vi "motioncontroller.vi"(3 "Error in x":errorcluster, 5 "VISA IN x":refnum<visa-resource-name>) -> (0 "Error out x":errorcluster, 2 "VISA OUT x":refnum<visa-resource-name>)   [LabVIEW 2016]
uses:
  <vilib>/Instr/_visa.llb/VISA Flush IO Buffer Mask.ctl
  <vilib>/Instr/_visa.llb/VISA Configure Serial Port (Instr).vi
panel:
  in  "Dy (mm)":dbl
  in  "Dx (mm)":dbl
  in  "y (mm)":dbl
  in  "x (mm)":dbl
  out "string to y (hex)":string
  in  "command to y":string
  out "VISA OUT y":refnum<visa-resource-name>
  out "Error out y":errorcluster
  out "answer from y (hex)":string
  in  "VISA IN y":refnum<visa-resource-name>
  in  "Error in y":errorcluster
  out "string to x (hex)":string
  in  "command to x":string
  in  "SHIFT":bool
  in  "MOVE":bool
  out "answer from x (hex)":string
  in  "SEND":bool
  in  "EXIT":bool
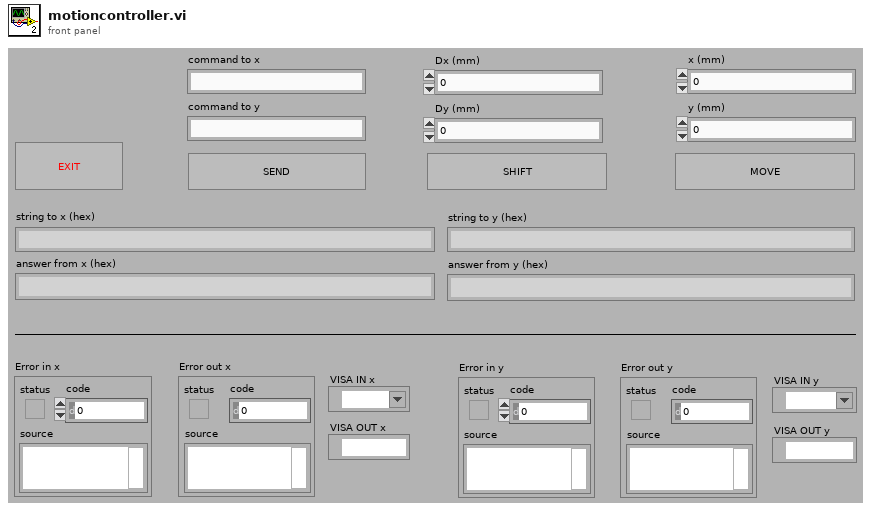
[diagram p1: front panel]
types:
  T1 = typedef "VISA Flush IO Buffer Mask.ctl" = u16
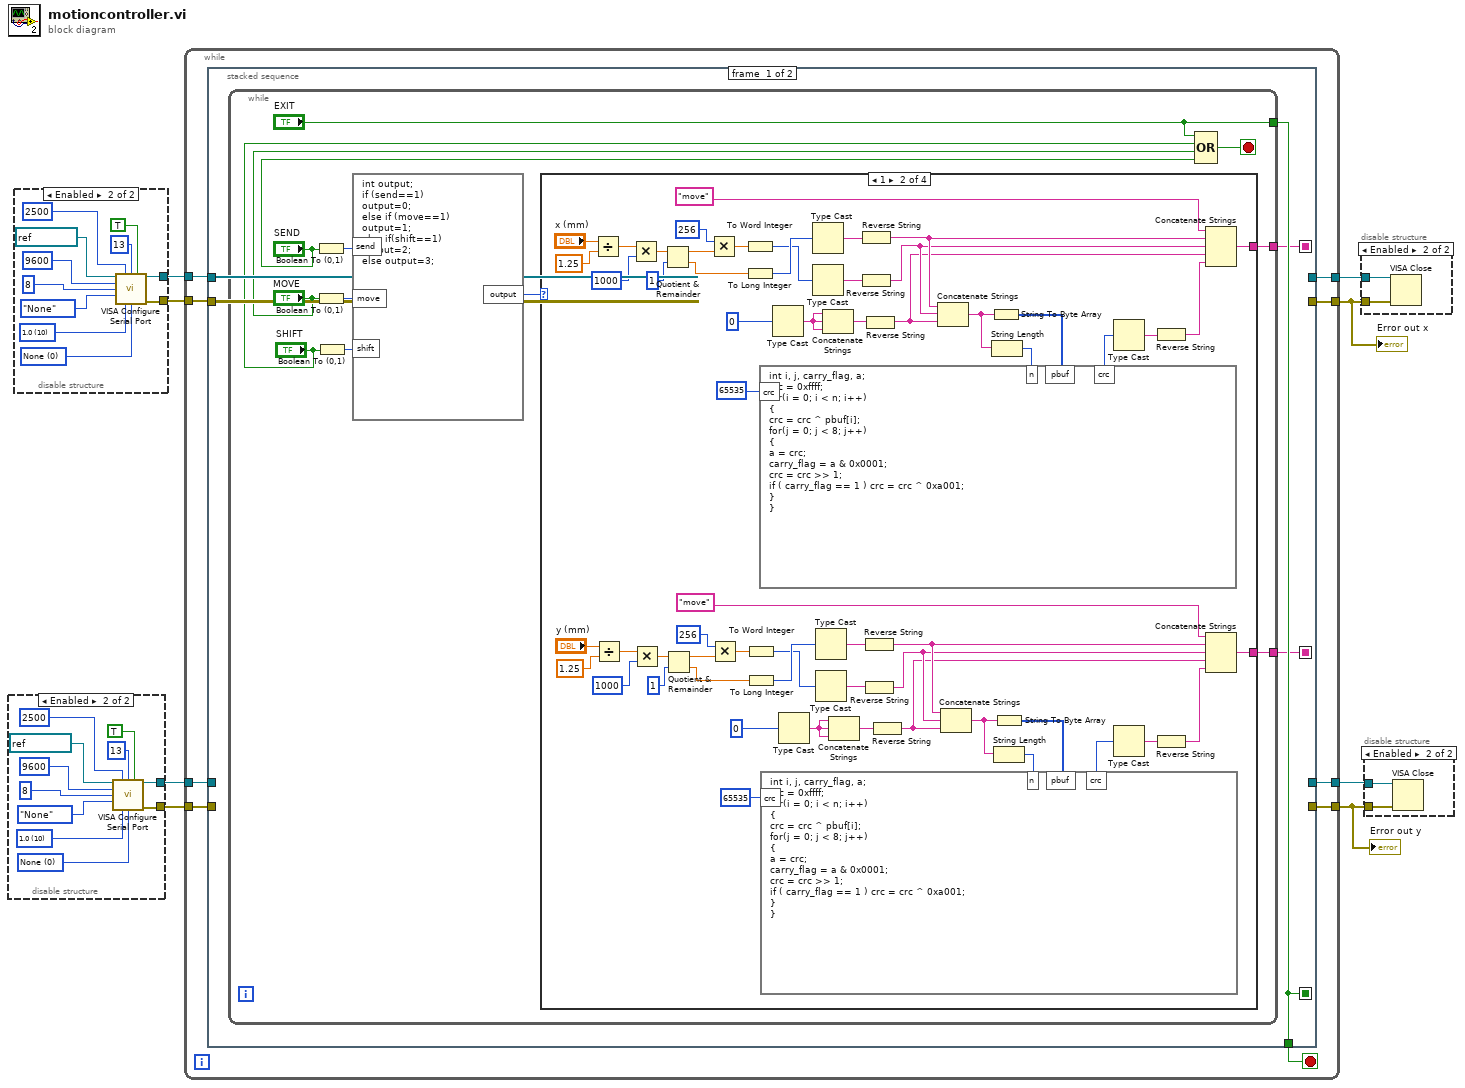
[diagram p0: block diagram]
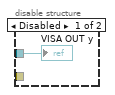
[diagram p2: hidden frame]
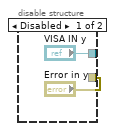
[diagram p3: hidden frame]
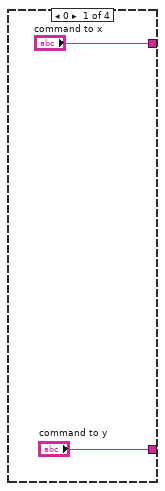
[diagram p4: hidden frame]
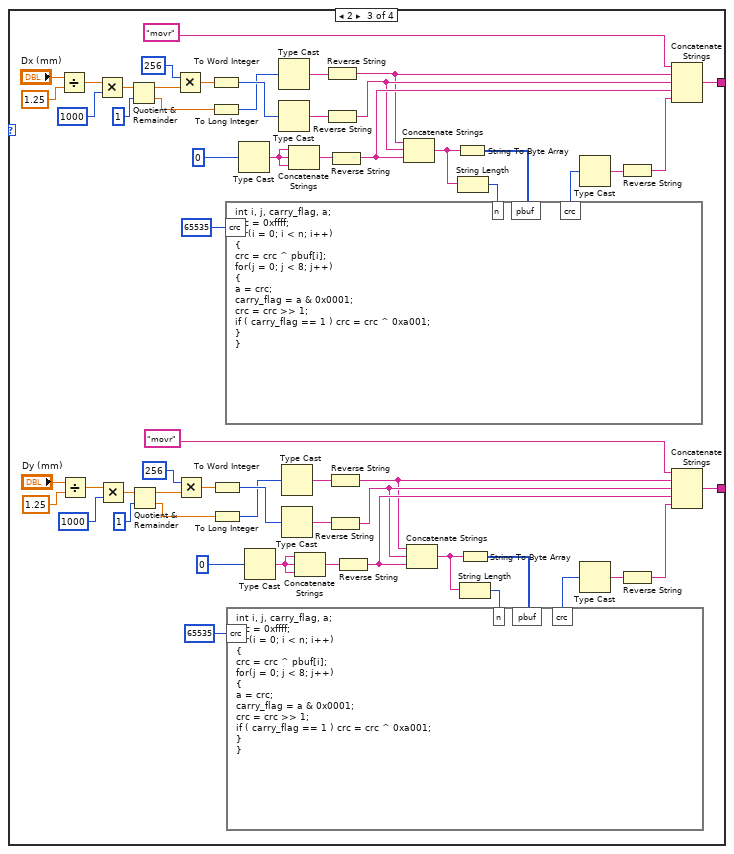
[diagram p5: hidden frame]
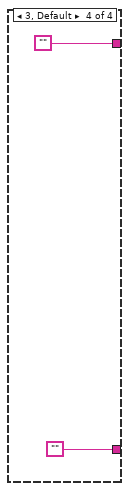
[diagram p6: hidden frame]
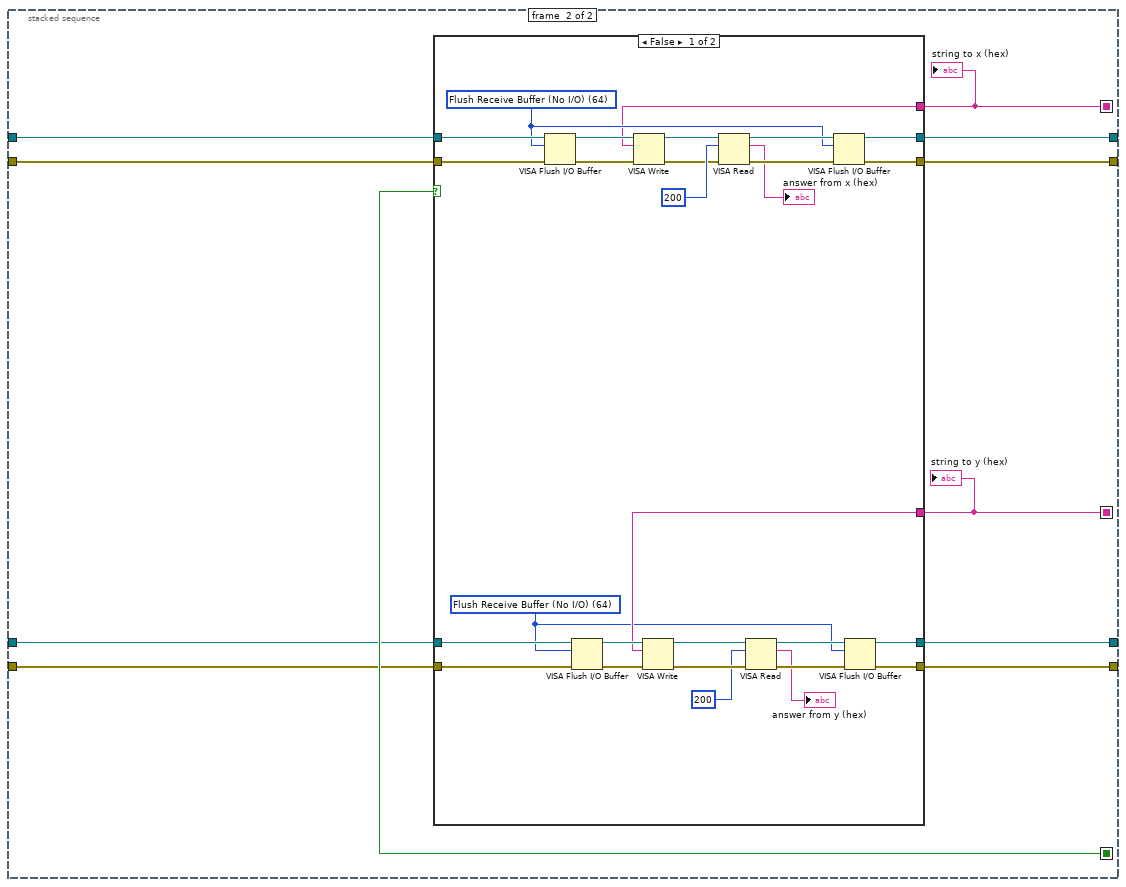
[diagram p7: hidden frame]
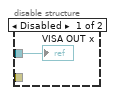
[diagram p9: hidden frame]
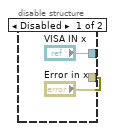
[diagram p10: hidden frame]
diagram:
  n1 = disable-structure shown="Enabled" {
    disable-tunnel: ["VISA IN y" w13] -> w6
    disable-tunnel: ["Error in y" w12] -> w5
    frame Disabled {
    }
    frame Enabled {
      w18 = u16 0 items=["None", "XON/XOFF", "RTS/CTS", "XON/XOFF & RTS/CTS", "DTR/DSR", "XON/XOFF & DTR/DSR"] ("flow control (0:none)")
      w17 = u16 10 items=["1.0"=10, "1.5"=15, "2.0"=20] ("stop bits (10: 1 bit)")
      n2 = call-poly "VISA Configure Serial Port"("VISA resource name"=refnum<visa-resource-name> "COM4" ("VISA resource name y"), "timeout (10sec)"=u32 2500, "termination char\n(0xA = '\\n' = LF)"=u8 13 ("termination char\n(0xA = '\\n' = LF)"), "Enable Termination\nChar (T)"=TRUE ("Enable Termination\nChar (T)"), "baud rate (9600)"=u32 9600, "data bits (8)"=u16 8, "parity (0:none)"=enum16{"None", "Odd", "Even", "Mark", "Space"}."None", "stop bits (10: 1 bit)"=w17, "flow control (0:none)"=w18) -> ("VISA resource name out"=w13:refnum<visa-resource-name>, "error out"=w12:errorcluster)  [unwired: 1 in, 4 out]
    }
  }
  n3 = disable-structure shown="Enabled" {
    disable-tunnel: ["VISA IN x" w26] -> w8
    disable-tunnel: ["Error in x" w25] -> w7
    frame Disabled {
    }
    frame Enabled {
      w31 = u16 0 items=["None", "XON/XOFF", "RTS/CTS", "XON/XOFF & RTS/CTS", "DTR/DSR", "XON/XOFF & DTR/DSR"] ("flow control (0:none)")
      w30 = u16 10 items=["1.0"=10, "1.5"=15, "2.0"=20] ("stop bits (10: 1 bit)")
      n4 = call-poly "VISA Configure Serial Port"("VISA resource name"=refnum<visa-resource-name> "COM3" ("VISA resource name x"), "timeout (10sec)"=u32 2500, "termination char\n(0xA = '\\n' = LF)"=u8 13 ("termination char\n(0xA = '\\n' = LF)"), "Enable Termination\nChar (T)"=TRUE ("Enable Termination\nChar (T)"), "baud rate (9600)"=u32 9600, "data bits (8)"=u16 8, "parity (0:none)"=enum16{"None", "Odd", "Even", "Mark", "Space"}."None", "stop bits (10: 1 bit)"=w30, "flow control (0:none)"=w31) -> ("VISA resource name out"=w26:refnum<visa-resource-name>, "error out"=w25:errorcluster)  [unwired: 1 in, 4 out]
    }
  }
  n5 = while {
    tunnel: w8 -> [w43]
    tunnel: w7 -> [w42]
    tunnel: w6 -> [w40]
    tunnel: w5 -> [w39]
    tunnel: [w38] -> w4
    tunnel: [w37] -> w3
    tunnel: [w36] -> w1
    tunnel: [w35] -> w2
    stop <- w41 stop-if-true
    n6 = stacked-sequence {
      seq-local: [w46 _] -> [_ w184]
      seq-local: [w44 _] -> [_ w178]
      seq-local: [w45 _] -> [_ w179]
      tunnel: [_ w188] -> w36
      tunnel: w43 -> [_ w187]
      tunnel: w42 -> [_ w186]
      tunnel: [_ w185] -> w35
      tunnel: [w46 _] -> w41
      tunnel: w40 -> [_ w183]
      tunnel: w39 -> [_ w182]
      tunnel: [_ w181] -> w38
      tunnel: [_ w180] -> w37
      frame #0 {
        n7 = while {
          tunnel: ["EXIT"] -> w46
          tunnel: [w48] -> w44
          tunnel: [w47] -> w45
          stop <- w53 stop-if-true
          n8 = Boolean To (0,1)(Boolean="SEND") -> (0, 1=w56:i16)
          n9 = Boolean To (0,1)(Boolean="MOVE") -> (0, 1=w55:i16)
          n10 = Boolean To (0,1)(Boolean="SHIFT") -> (0, 1=w54:i16)
          n11 = formula code="int output;\nif (send==1)\noutput=0;\nelse if (move==1)\noutput=1;\nelse if(shift==1)\noutput=2;\nelse output=3;"("send"=w56, "move"=w55, "shift"=w54) -> ("output"=w57:i32)
          n12 = case shown="1" w57 {
            tunnel: ["command to x" w60 w119 ""] -> w48
            tunnel: ["command to y" w61 w118 ""] -> w47
            frame 0 {
            }
            frame 1 {
              n13 = Divide(x="x (mm)", y=1.25) -> (x/y=w84:dbl)
              n14 = Divide(x="y (mm)", y=1.25) -> (x/y=w73:dbl)
              n15 = Multiply(x=w84, y=1000) -> (x*y=w82:dbl)
              n16 = Multiply(x=w73, y=1000) -> (x*y=w71:dbl)
              n17 = Quotient & Remainder(x=w82, y=1) -> (x-y*floor(x/y)=w80:dbl, floor(x/y)=w78:dbl)
              n18 = Quotient & Remainder(x=w71, y=1) -> (x-y*floor(x/y)=w69:dbl, floor(x/y)=w67:dbl)
              n19 = Multiply(x=256, y=w80) -> (x*y=w76:dbl)
              n20 = Multiply(x=256, y=w69) -> (x*y=w66:dbl)
              n21 = To Word Integer(number=w76) -> (16bit integer=w75:i16)
              n22 = To Long Integer(number=w78) -> (32bit integer=w77:i32)
              n23 = To Word Integer(number=w66) -> (16bit integer=w64:i16)
              n24 = To Long Integer(number=w67) -> (32bit integer=w65:i32)
              n25 = Type Cast(x=u16 0) -> (*(type *) &x=w111:string)  [unwired: 1 in]
              n26 = Type Cast(x=u16 0) -> (*(type *) &x=w104:string)  [unwired: 1 in]
              n27 = Type Cast(x=w77) -> (*(type *) &x=w101:string)  [unwired: 1 in]
              n28 = Type Cast(x=w75) -> (*(type *) &x=w99:string)  [unwired: 1 in]
              n29 = Type Cast(x=w65) -> (*(type *) &x=w91:string)  [unwired: 1 in]
              n30 = Type Cast(x=w64) -> (*(type *) &x=w89:string)  [unwired: 1 in]
              n31 = Concatenate Strings(w111, w111, w111) -> (w97:string)
              n32 = Concatenate Strings(w104, w104, w104) -> (w87:string)
              n33 = Reverse String(1:w101) -> (0:w100:string)
              n34 = Reverse String(1:w99) -> (0:w98:string)
              n35 = Reverse String(1:w91) -> (0:w90:string)
              n36 = Reverse String(1:w89) -> (0:w88:string)
              n37 = Reverse String(1:w97) -> (0:w96:string)
              n38 = Reverse String(1:w87) -> (0:w86:string)
              n39 = Concatenate Strings(w100, w98, w96) -> (w116:string)
              n40 = Concatenate Strings(w90, w88, w86) -> (w109:string)
              n41 = String To Byte Array(string=w116) -> (unsigned byte array=w117:u8[])
              n42 = String Length(string=w116) -> (length=w115:i32)
              n43 = formula code="int i, j, carry_flag, a;\ncrc = 0xffff;\nfor(i = 0; i < n; i++)\n{\ncrc = crc ^ pbuf[i];\nfor(j = 0; j < 8; j++)\n{\na = crc;\ncarry_flag = a & 0x0001;\ncrc = crc >> 1;\nif ( carry_flag == 1 ) crc = crc ^ 0xa001;\n}\n}"("n"=w115, "pbuf"=w117, "crc"=u16 65535) -> ("crc"=w103:u16)
              n44 = String To Byte Array(string=w109) -> (unsigned byte array=w110:u8[])
              n45 = String Length(string=w109) -> (length=w108:i32)
              n46 = formula code="int i, j, carry_flag, a;\ncrc = 0xffff;\nfor(i = 0; i < n; i++)\n{\ncrc = crc ^ pbuf[i];\nfor(j = 0; j < 8; j++)\n{\na = crc;\ncarry_flag = a & 0x0001;\ncrc = crc >> 1;\nif ( carry_flag == 1 ) crc = crc ^ 0xa001;\n}\n}"("n"=w108, "pbuf"=w110, "crc"=u16 65535) -> ("crc"=w102:u16)
              n47 = Type Cast(x=w103) -> (*(type *) &x=w93:string)  [unwired: 1 in]
              n48 = Type Cast(x=w102) -> (*(type *) &x=w95:string)  [unwired: 1 in]
              n49 = Reverse String(1:w93) -> (0:w92:string)
              n50 = Reverse String(1:w95) -> (0:w94:string)
              n51 = Concatenate Strings("move" ("move to"), w100, w98, w96, w92) -> (w60:string)
              n52 = Concatenate Strings("move" ("move to"), w90, w88, w86, w94) -> (w61:string)
            }
            frame 2 {
              n53 = Divide(x="Dx (mm)", y=1.25) -> (x/y=w153:dbl)
              n54 = Divide(x="Dy (mm)", y=1.25) -> (x/y=w164:dbl)
              n55 = Multiply(x=w153, y=1000) -> (x*y=w155:dbl)
              n56 = Multiply(x=w164, y=1000) -> (x*y=w166:dbl)
              n57 = Quotient & Remainder(x=w155, y=1) -> (x-y*floor(x/y)=w157:dbl, floor(x/y)=w159:dbl)
              n58 = Quotient & Remainder(x=w166, y=1) -> (x-y*floor(x/y)=w168:dbl, floor(x/y)=w170:dbl)
              n59 = Multiply(x=256, y=w157) -> (x*y=w161:dbl)
              n60 = Multiply(x=256, y=w168) -> (x*y=w171:dbl)
              n61 = To Word Integer(number=w161) -> (16bit integer=w162:i16)
              n62 = To Long Integer(number=w159) -> (32bit integer=w160:i32)
              n63 = To Word Integer(number=w171) -> (16bit integer=w173:i16)
              n64 = To Long Integer(number=w170) -> (32bit integer=w172:i32)
              n65 = Type Cast(x=u16 0) -> (*(type *) &x=w126:string)  [unwired: 1 in]
              n66 = Type Cast(x=u16 0) -> (*(type *) &x=w133:string)  [unwired: 1 in]
              n67 = Type Cast(x=w160) -> (*(type *) &x=w136:string)  [unwired: 1 in]
              n68 = Type Cast(x=w162) -> (*(type *) &x=w138:string)  [unwired: 1 in]
              n69 = Type Cast(x=w172) -> (*(type *) &x=w146:string)  [unwired: 1 in]
              n70 = Type Cast(x=w173) -> (*(type *) &x=w148:string)  [unwired: 1 in]
              n71 = Concatenate Strings(w126, w126, w126) -> (w140:string)
              n72 = Concatenate Strings(w133, w133, w133) -> (w150:string)
              n73 = Reverse String(1:w136) -> (0:w137:string)
              n74 = Reverse String(1:w138) -> (0:w139:string)
              n75 = Reverse String(1:w146) -> (0:w147:string)
              n76 = Reverse String(1:w148) -> (0:w149:string)
              n77 = Reverse String(1:w140) -> (0:w141:string)
              n78 = Reverse String(1:w150) -> (0:w151:string)
              n79 = Concatenate Strings(w137, w139, w141) -> (w121:string)
              n80 = Concatenate Strings(w147, w149, w151) -> (w128:string)
              n81 = String To Byte Array(string=w121) -> (unsigned byte array=w120:u8[])
              n82 = String Length(string=w121) -> (length=w122:i32)
              n83 = formula code="int i, j, carry_flag, a;\ncrc = 0xffff;\nfor(i = 0; i < n; i++)\n{\ncrc = crc ^ pbuf[i];\nfor(j = 0; j < 8; j++)\n{\na = crc;\ncarry_flag = a & 0x0001;\ncrc = crc >> 1;\nif ( carry_flag == 1 ) crc = crc ^ 0xa001;\n}\n}"("n"=w122, "pbuf"=w120, "crc"=u16 65535) -> ("crc"=w134:u16)
              n84 = String To Byte Array(string=w128) -> (unsigned byte array=w127:u8[])
              n85 = String Length(string=w128) -> (length=w129:i32)
              n86 = formula code="int i, j, carry_flag, a;\ncrc = 0xffff;\nfor(i = 0; i < n; i++)\n{\ncrc = crc ^ pbuf[i];\nfor(j = 0; j < 8; j++)\n{\na = crc;\ncarry_flag = a & 0x0001;\ncrc = crc >> 1;\nif ( carry_flag == 1 ) crc = crc ^ 0xa001;\n}\n}"("n"=w129, "pbuf"=w127, "crc"=u16 65535) -> ("crc"=w135:u16)
              n87 = Type Cast(x=w134) -> (*(type *) &x=w144:string)  [unwired: 1 in]
              n88 = Type Cast(x=w135) -> (*(type *) &x=w142:string)  [unwired: 1 in]
              n89 = Reverse String(1:w144) -> (0:w145:string)
              n90 = Reverse String(1:w142) -> (0:w143:string)
              n91 = Concatenate Strings("movr" ("move to"), w137, w139, w141, w145) -> (w119:string)
              n92 = Concatenate Strings("movr" ("move to"), w147, w149, w151, w143) -> (w118:string)
            }
            frame 3, Default {
            }
          }
          n93 = Compound Arithmetic op=OR("EXIT", "SHIFT", "MOVE", "SEND") -> (w53:bool)
        }
      }
      frame #1 {
        n94 = case shown="False" w184 {
          tunnel: [w213 w220] -> w188
          tunnel: w187 -> [w211 w220]
          tunnel: w186 -> [w209 w219]
          tunnel: [w205 w219] -> w185
          tunnel: w178 -> [w189 _]
          tunnel: w183 -> [w198 w218]
          tunnel: w182 -> [w197 w217]
          tunnel: [w196 w218] -> w181
          tunnel: [w195 w217] -> w180
          tunnel: w179 -> [w191 _]
          frame False {
            w190 = T1 64 items=["Flush Receive Buffer"=16, "Write Transmit Buffer to Device"=32, "Flush Receive Buffer (No I/O)"=64, "Flush Transmit Buffer"=128] ("Mask")
            w210 = T1 64 items=["Flush Receive Buffer"=16, "Write Transmit Buffer to Device"=32, "Flush Receive Buffer (No I/O)"=64, "Flush Transmit Buffer"=128] ("Mask")
            n95 = VISA Flush I/O Buffer(VISA resource name=w211, mask (16)=w210, error in (no error)=w209) -> (VISA resource name out=w212:refnum<visa-resource-name>, error out=w208:errorcluster)
            n96 = VISA Flush I/O Buffer(VISA resource name=w198, mask (16)=w190, error in (no error)=w197) -> (VISA resource name out=w201:refnum<visa-resource-name>, error out=w202:errorcluster)
            n97 = VISA Write(VISA resource name=w212, write buffer=w189, error in (no error)=w208) -> (VISA resource name out=w215:refnum<visa-resource-name>, error out=w207:errorcluster)  [unwired: 1 out]
            n98 = VISA Write(VISA resource name=w201, write buffer=w191, error in (no error)=w202) -> (VISA resource name out=w199:refnum<visa-resource-name>, error out=w203:errorcluster)  [unwired: 1 out]
            n99 = VISA Read(VISA resource name=w215, byte count=u32 200, error in (no error)=w207) -> (VISA resource name out=w214:refnum<visa-resource-name>, read buffer=→"answer from x (hex)":string, error out=w206:errorcluster)  [unwired: 1 out]
            n100 = VISA Read(VISA resource name=w199, byte count=u32 200, error in (no error)=w203) -> (VISA resource name out=w200:refnum<visa-resource-name>, read buffer=→"answer from y (hex)":string, error out=w204:errorcluster)  [unwired: 1 out]
            n101 = VISA Flush I/O Buffer(VISA resource name=w214, mask (16)=w210, error in (no error)=w206) -> (VISA resource name out=w213:refnum<visa-resource-name>, error out=w205:errorcluster)
            n102 = VISA Flush I/O Buffer(VISA resource name=w200, mask (16)=w190, error in (no error)=w204) -> (VISA resource name out=w196:refnum<visa-resource-name>, error out=w195:errorcluster)
          }
          frame True {
          }
        }
        "string to x (hex)" <- w178
        "string to y (hex)" <- w179
      }
    }
  }
  "Error out x" <- w2
  "Error out y" <- w3
  n103 = disable-structure shown="Enabled" {
    disable-tunnel: w2 -> [_ w223]
    disable-tunnel: w1 -> [w221 w222]
    frame Disabled {
      "VISA OUT x" <- w221
    }
    frame Enabled {
      n104 = VISA Close(VISA resource name=w222, error in (no error)=w223) -> ()  [unwired: 1 out]
    }
  }
  n105 = disable-structure shown="Enabled" {
    disable-tunnel: w4 -> [w224 w226]
    disable-tunnel: w3 -> [_ w225]
    frame Disabled {
      "VISA OUT y" <- w224
    }
    frame Enabled {
      n106 = VISA Close(VISA resource name=w226, error in (no error)=w225) -> ()  [unwired: 1 out]
    }
  }
